vi "GetCMDLine.vi"(8 "error in (no error)":errorcluster, 11 "application in":refnum<class "application.lvclass">) -> (0 "error out":errorcluster, 3 "application out":refnum<class "application.lvclass">)   [LabVIEW 2017, in "application.lvlib" / "application.lvclass"]
uses:
  application.lvclass
  application.lvclass/application.ctl
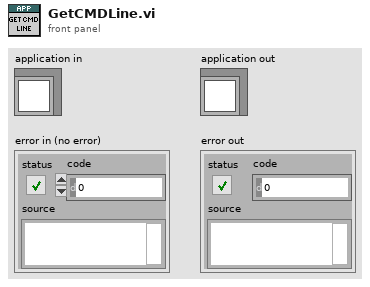
[diagram p1: front panel]
types:
  T1 = typedef "application.lvlib/application.lvclass/DEF-LabVIEW INFO.ctl" = cluster{"Version":string, "Path":path}
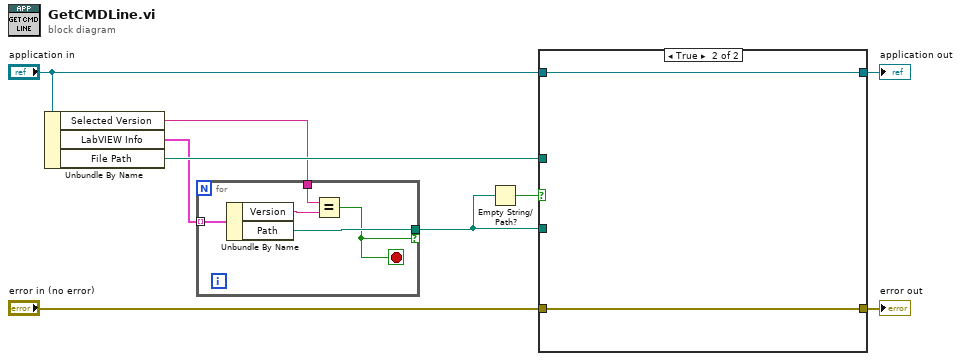
[diagram p0: block diagram]
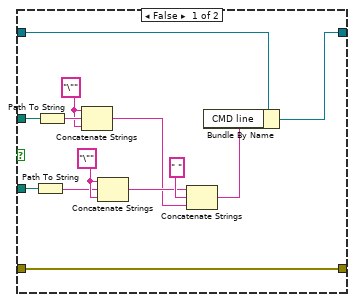
[diagram p2: hidden frame]
diagram:
  n1 = Unbundle By Name("application in") -> ("Selected Version"=w5:string, "LabVIEW Info"=w6:T1[], "File Path"=w7:path)
  n2 = for {
    tunnel: w6 -> [w14] mode=indexing
    tunnel: [w12] -> w3 if=w10
    tunnel: w5 -> [w11]
    stop <- w10 stop-if-true
    n3 = Unbundle By Name(w14) -> ("Version"=w13:string, "Path"=w12:path)
    n4 = Equal?(x=w11, y=w13) -> (x = y?=w10:bool)
  }
  n5 = Empty String/Path?(string/path=w3) -> (empty?=w4:bool)
  n6 = case shown="True" w4 {
    tunnel: "error in (no error)" -> [w15 w29]
    tunnel: w3 -> [w27 _]
    tunnel: [w15 w29] -> w2
    tunnel: w7 -> [w19 _]
    tunnel: "application in" -> [w18 w28]
    tunnel: [w17 w28] -> w9
    frame False {
      w24 = "\"" ("string")
      w25 = "\"" ("string")
      n7 = Path To String(path=w27) -> (string=w23:string)
      n8 = Path To String(path=w19) -> (string=w26:string)
      n9 = Concatenate Strings(w25, w26, w25) -> (w20:string)
      n10 = Concatenate Strings(w24, w23, w24) -> (w21:string)
      n11 = Concatenate Strings(w21, " " ("string"), w20) -> (w16:string)
      n12 = Bundle By Name(cluster=w18, "CMD line"=w16) -> (w17:refnum<class "application.lvclass">)
    }
    frame True {
    }
  }
  "application out" <- w9
  "error out" <- w2
